vi "Gannt Chart Crossover.vi"(8 "error in (no error)":errorcluster, 11 "GA in":refnum<class "GA.lvclass">) -> (0 "error out":errorcluster, 3 "GA out":refnum<class "GA.lvclass">)   [LabVIEW 2013, in "GA.lvclass"]
uses:
  GA.lvclass
  GA.lvclass/GA.ctl
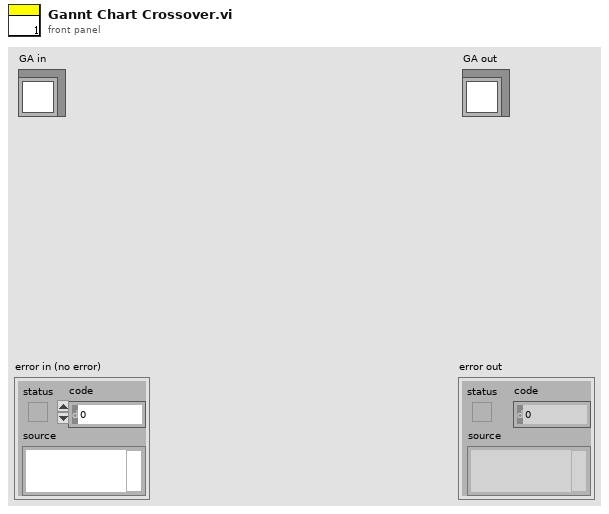
[diagram p1: front panel]
types:
  T1 = typedef "Solution_GA.ctl" = cluster{"Schedule":u16[], "Fitness":u16, "Fitness Valid?":bool}
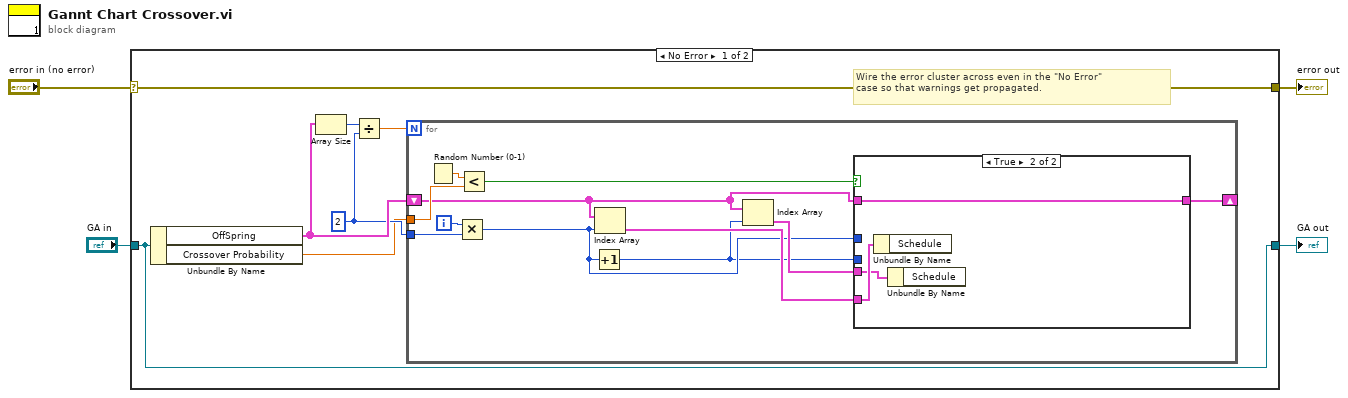
[diagram p0: block diagram]
diagram:
  n1 = case shown="No Error" "error in (no error)" {
    selector: "error in (no error)" -> [w11 w28]
    tunnel: [w11 w28] -> w3
    tunnel: [w5 w27] -> w1
    tunnel: "GA in" -> [w5 w27]
    frame No Error {
      w7 = 2 ("y")
      # "Wire the error cluster across even in the \"No Error\"\ncase so that warnings get propagated."
      n2 = Unbundle By Name(w5) -> ("OffSpring"=w8:T1[], "Crossover Probability"=w6:dbl)
      n3 = Array Size(array=w8) -> (size(s)=w10:i32)
      n4 = Divide(x=w10, y=w7) -> (x/y=w9:dbl)
      n5 = for {
        N: w9 -> [_]
        tunnel: w7 -> [w22]
        tunnel: w6 -> [w19]
        shift-right: [w12] -> _
        shift-left: w8 -> [w15]
        i -> [w21]
        n6 = Random Number (0-1)() -> (number: 0 to 1=w20:dbl)
        n7 = Multiply(x=w21, y=w22) -> (x*y=w14:i32)
        n8 = Less?(x=w20, y=w19) -> (x < y?=w18:bool)
        n9 = Increment(x=w14) -> (x+1=w13:i32)
        n10 = Index Array(array=w15, index=w14) -> (element=w17:T1)
        n11 = Index Array(array=w15, index=w13) -> (element=w16:T1)
        n12 = case shown="True" w18 {
          tunnel: w17 -> [_ w25]
          tunnel: w16 -> [_ w24]
          tunnel: w15 -> [w23 w26]
          tunnel: w14 -> [_ _]
          tunnel: w13 -> [_ _]
          tunnel: [w23 w26] -> w12
          frame False {
          }
          frame True {
            n13 = Unbundle By Name(w25) -> ()  [unwired: 1 out]
            n14 = Unbundle By Name(w24) -> ()  [unwired: 1 out]
          }
        }
      }
    }
    frame Error {
    }
  }
  "error out" <- w3
  "GA out" <- w1
